vi "obstacle2.vi"(9 "Numeric":dbl, 10 "f":i32, 11 "Position in":T1) -> (0 "deliver":bool, 3 "Position out":T1)   [LabVIEW 2014]
uses:
  <vilib>/Utility/miscctls.llb/LVPositionTypeDef.ctl
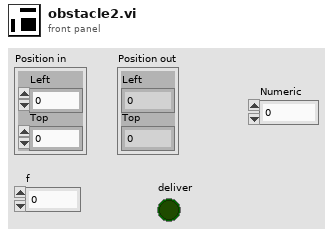
[diagram p1: front panel]
types:
  T1 = typedef "LVPositionTypeDef.ctl" = cluster{"Left":i32, "Top":i32}
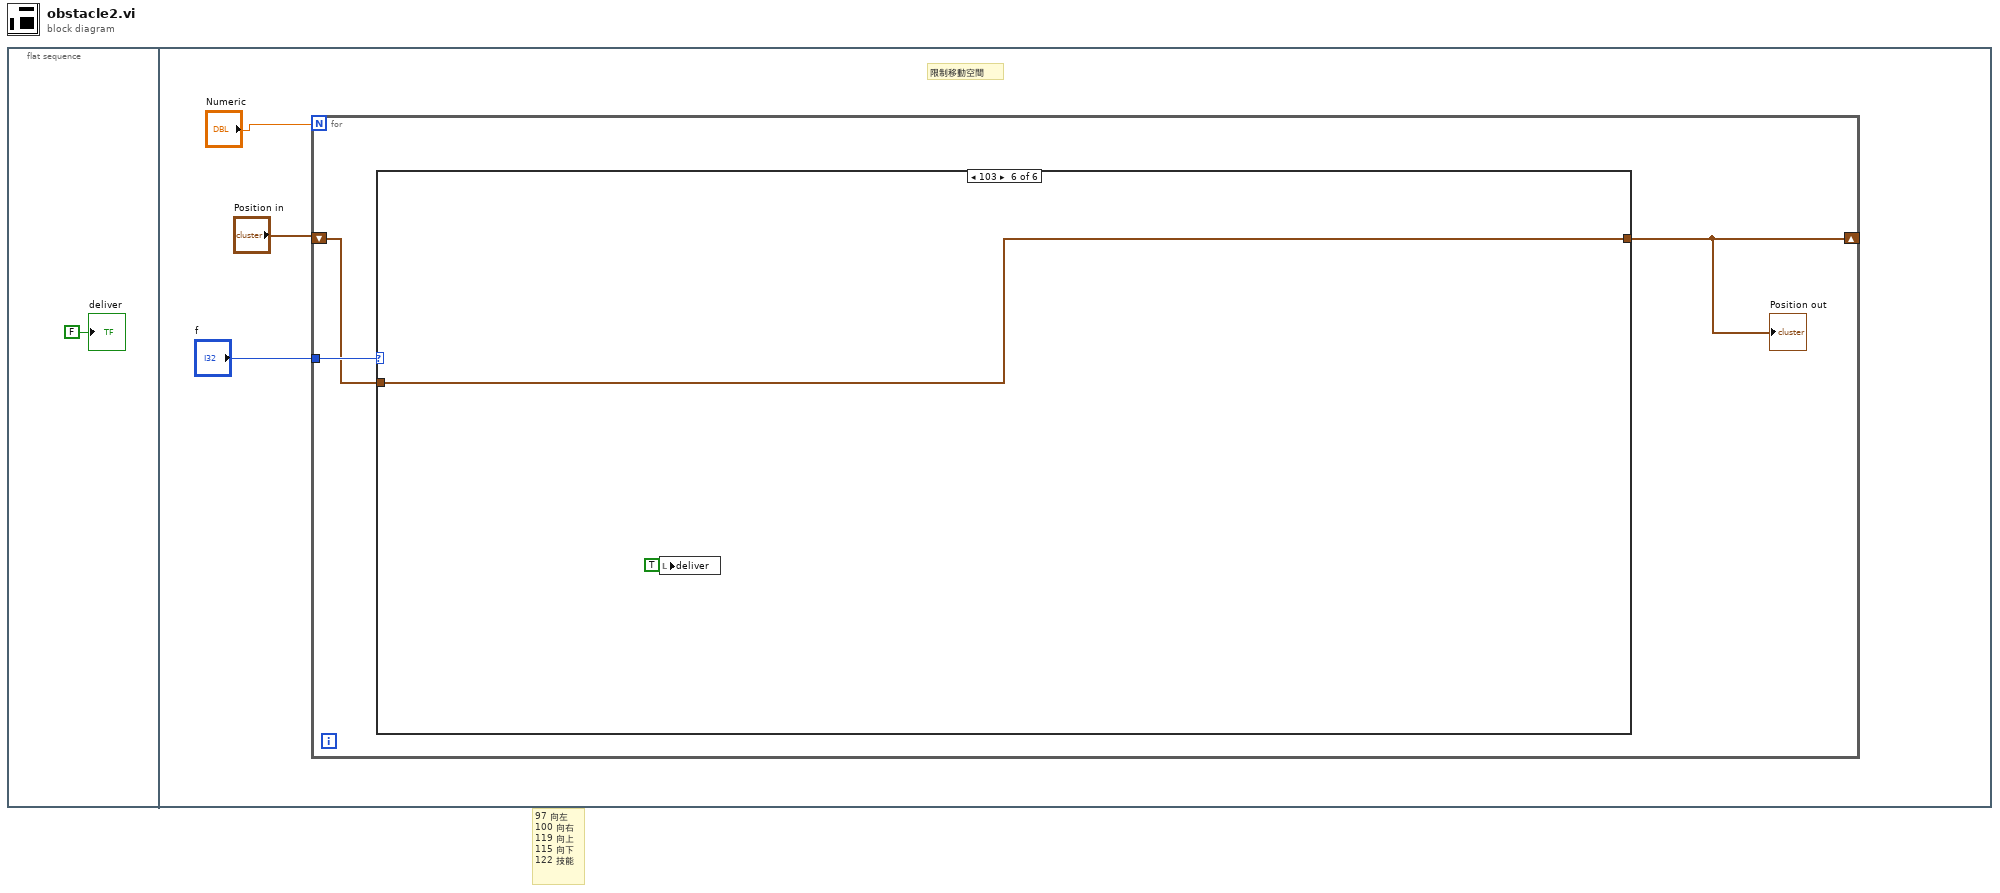
[diagram p0: block diagram]
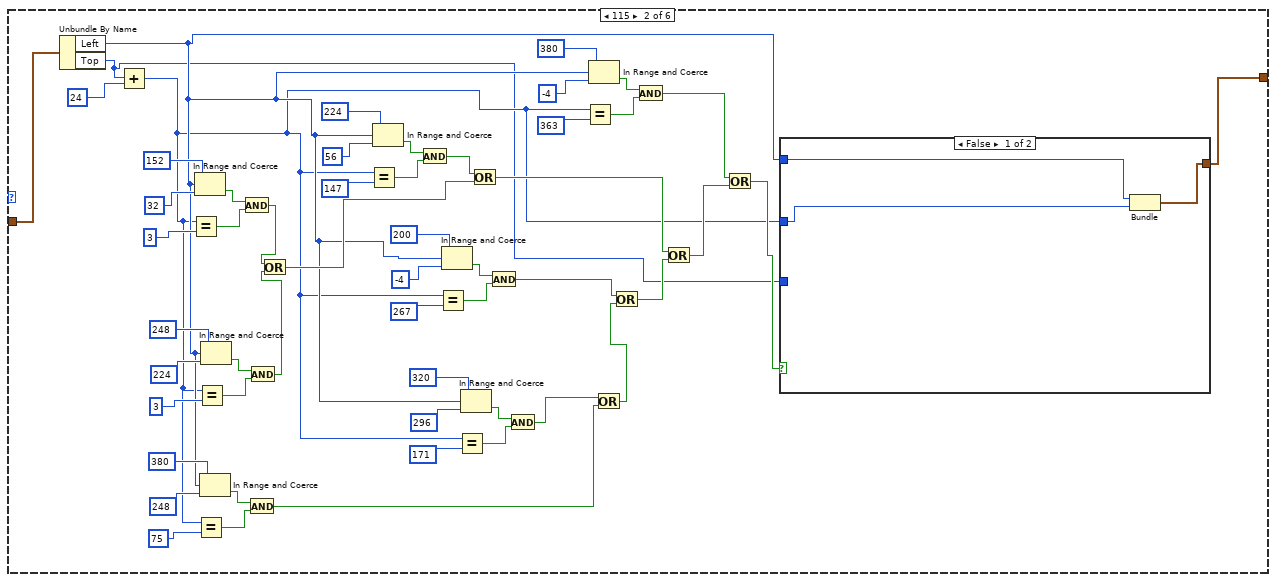
[diagram p3: hidden frame]
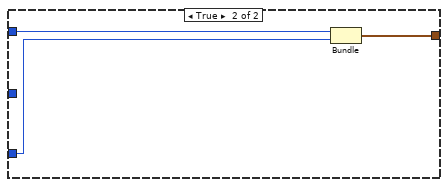
[diagram p4: hidden frame]
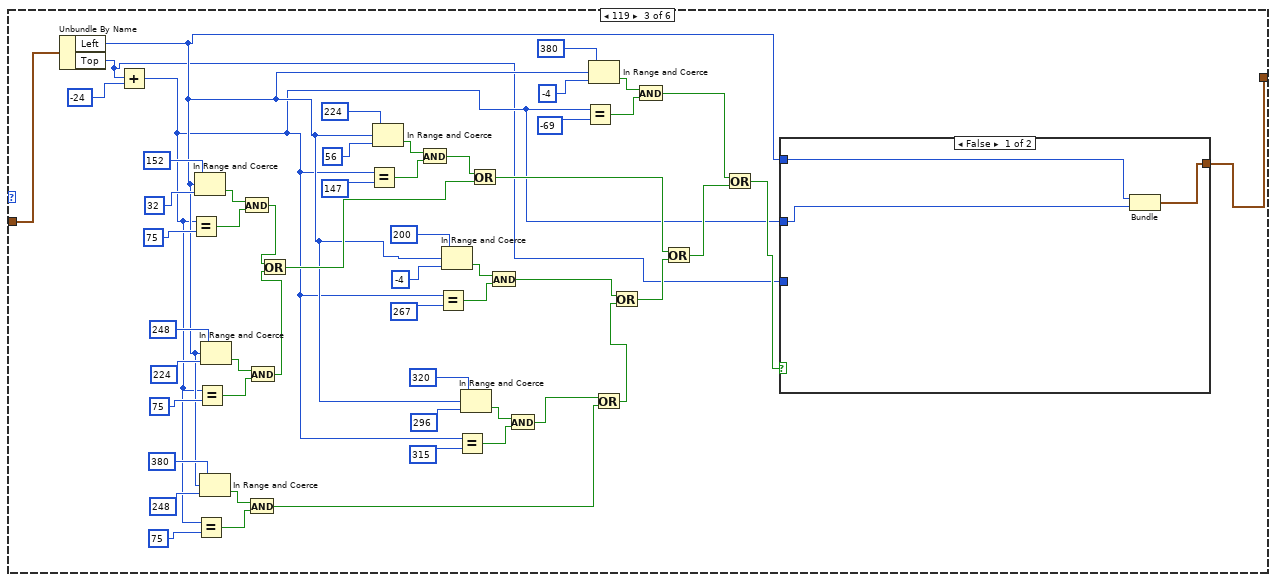
[diagram p5: hidden frame]
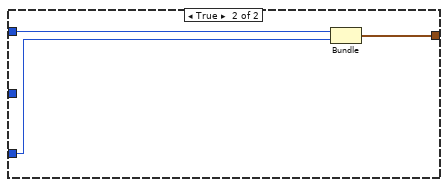
[diagram p6: hidden frame]
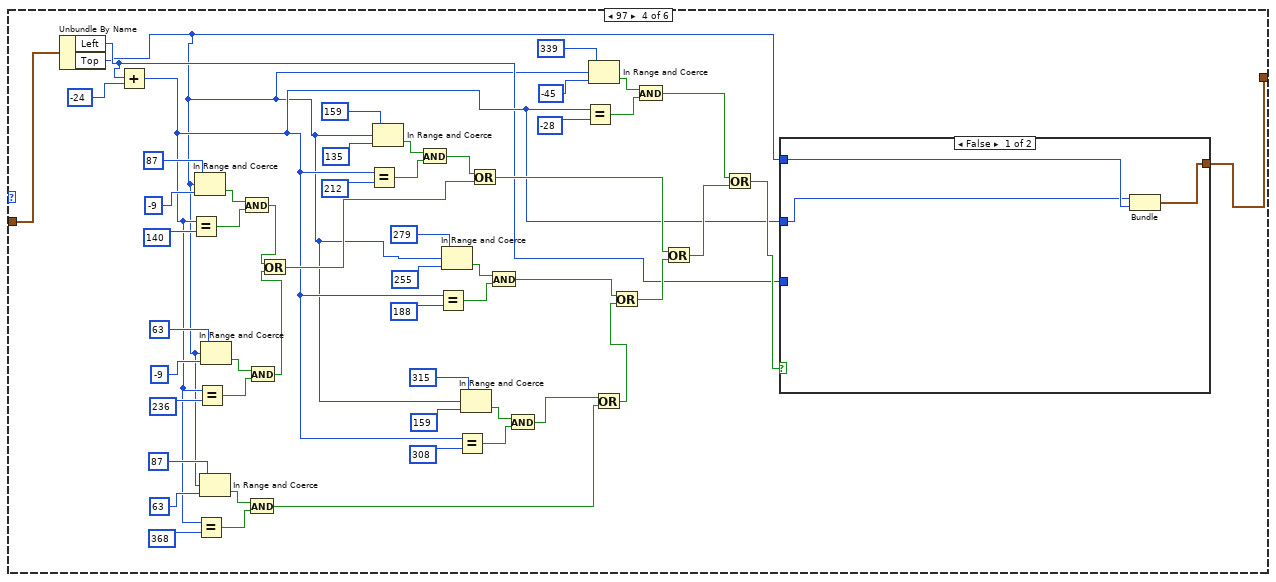
[diagram p7: hidden frame]
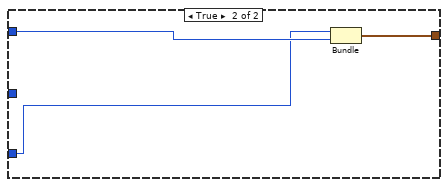
[diagram p8: hidden frame]
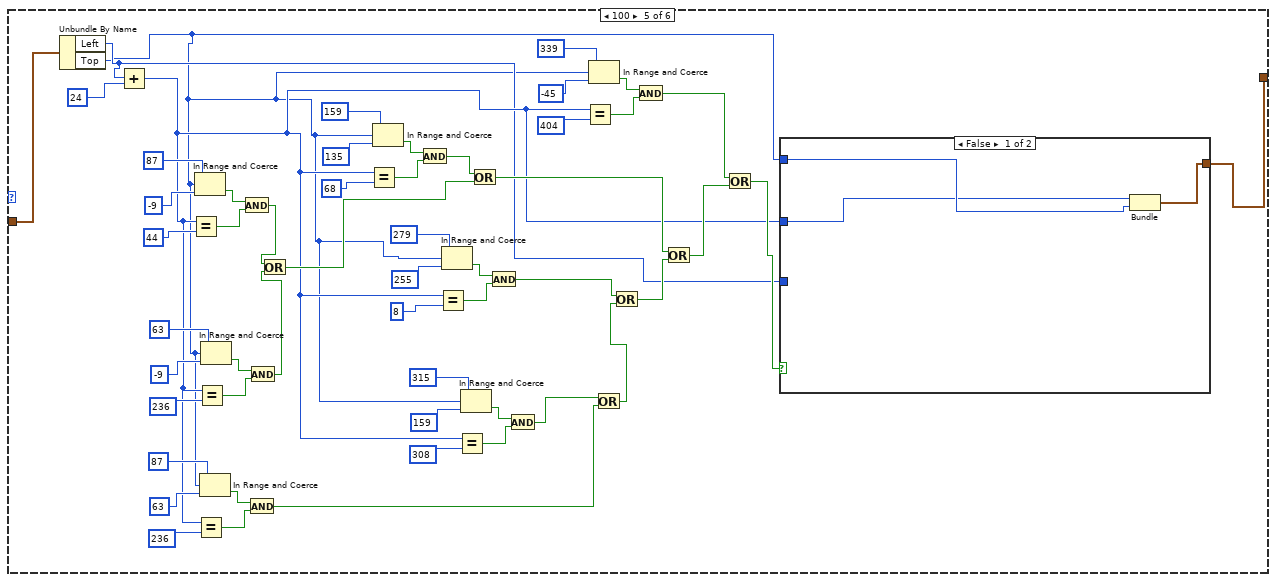
[diagram p9: hidden frame]
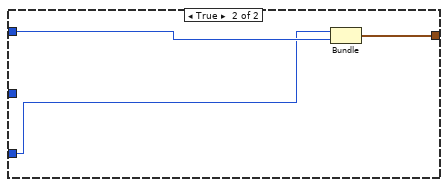
[diagram p10: hidden frame]
diagram:
  # "97 向左\n100 向右\n119 向上\n115 向下\n122 技能"
  n1 = flat-sequence {
    frame #0 {
      "deliver" <- FALSE ("skill")
    }
    frame #1 {
      # "限制移動空間"
      n2 = for {
        N: "Numeric" -> [_]
        tunnel: "f" -> [w7]
        shift-right: [w6] -> _
        shift-left: "Position in" -> [w5]
        n3 = case shown="103" w7 {
          tunnel: w5 -> [w8 w61 w121 w181 w241 w250]
          tunnel: [w8 w9 w120 w180 w240 w250] -> w6
          frame 0, Default {
          }
          frame 115 {
            n4 = Unbundle By Name(w61) -> ("Left"=w12:i32, "Top"=w10:i32)
            n5 = Add(x=w10, y=24) -> (x+y=w11:i32)
            n6 = Equal?(x=w11, y=3) -> (x = y?=w57:bool)
            n7 = In Range and Coerce(upper limit=152, x=w12, lower limit=32) -> (In Range?=w56:bool)  [unwired: 1 out]
            n8 = Equal?(x=w11, y=75) -> (x = y?=w47:bool)
            n9 = Equal?(x=w11, y=3) -> (x = y?=w52:bool)
            n10 = In Range and Coerce(upper limit=380, x=w12, lower limit=248) -> (In Range?=w46:bool)  [unwired: 1 out]
            n11 = In Range and Coerce(upper limit=248, x=w12, lower limit=224) -> (In Range?=w51:bool)  [unwired: 1 out]
            n12 = And(x=w56, y=w57) -> (x .and. y?=w30:bool)
            n13 = And(x=w46, y=w47) -> (x .and. y?=w26:bool)
            n14 = And(x=w51, y=w52) -> (x .and. y?=w29:bool)
            n15 = Or(x=w30, y=w29) -> (x .or. y?=w28:bool)
            n16 = Equal?(x=w11, y=147) -> (x = y?=w42:bool)
            n17 = In Range and Coerce(upper limit=224, x=w12, lower limit=56) -> (In Range?=w41:bool)  [unwired: 1 out]
            n18 = And(x=w41, y=w42) -> (x .and. y?=w27:bool)
            n19 = Equal?(x=w11, y=267) -> (x = y?=w37:bool)
            n20 = In Range and Coerce(upper limit=200, x=w12, lower limit=-4) -> (In Range?=w36:bool)  [unwired: 1 out]
            n21 = Equal?(x=w11, y=171) -> (x = y?=w32:bool)
            n22 = In Range and Coerce(upper limit=320, x=w12, lower limit=296) -> (In Range?=w31:bool)  [unwired: 1 out]
            n23 = Or(x=w27, y=w28) -> (x .or. y?=w21:bool)
            n24 = And(x=w36, y=w37) -> (x .and. y?=w24:bool)
            n25 = And(x=w31, y=w32) -> (x .and. y?=w25:bool)
            n26 = Equal?(x=w11, y=363) -> (x = y?=w17:bool)
            n27 = In Range and Coerce(upper limit=380, x=w12, lower limit=-4) -> (In Range?=w16:bool)  [unwired: 1 out]
            n28 = Or(x=w25, y=w26) -> (x .or. y?=w23:bool)
            n29 = Or(x=w24, y=w23) -> (x .or. y?=w22:bool)
            n30 = And(x=w16, y=w17) -> (x .and. y?=w15:bool)
            n31 = Or(x=w21, y=w22) -> (x .or. y?=w14:bool)
            n32 = Or(x=w15, y=w14) -> (x .or. y?=w13:bool)
            n33 = case shown="False" w13 {
              tunnel: w12 -> [w64 w67]
              tunnel: [w65 w68] -> w9
              tunnel: w11 -> [w63 _]
              tunnel: w10 -> [_ w66]
              frame False {
                n34 = Bundle("Left"=w64, w63) -> (w65:cluster{"Left":i32, i32})  [unwired: 1 in]
              }
              frame True {
                n35 = Bundle("Left"=w67, "Top"=w66) -> (w68:cluster{"Left":i32, "Top":i32})  [unwired: 1 in]
              }
            }
          }
          frame 119 {
            n36 = Unbundle By Name(w121) -> ("Left"=w71:i32, "Top"=w69:i32)
            n37 = Add(x=w69, y=-24) -> (x+y=w70:i32)
            n38 = Equal?(x=w70, y=75) -> (x = y?=w116:bool)
            n39 = In Range and Coerce(upper limit=152, x=w71, lower limit=32) -> (In Range?=w115:bool)  [unwired: 1 out]
            n40 = Equal?(x=w70, y=75) -> (x = y?=w106:bool)
            n41 = Equal?(x=w70, y=75) -> (x = y?=w111:bool)
            n42 = In Range and Coerce(upper limit=380, x=w71, lower limit=248) -> (In Range?=w105:bool)  [unwired: 1 out]
            n43 = In Range and Coerce(upper limit=248, x=w71, lower limit=224) -> (In Range?=w110:bool)  [unwired: 1 out]
            n44 = And(x=w115, y=w116) -> (x .and. y?=w89:bool)
            n45 = And(x=w105, y=w106) -> (x .and. y?=w85:bool)
            n46 = And(x=w110, y=w111) -> (x .and. y?=w88:bool)
            n47 = Or(x=w89, y=w88) -> (x .or. y?=w87:bool)
            n48 = Equal?(x=w70, y=147) -> (x = y?=w101:bool)
            n49 = In Range and Coerce(upper limit=224, x=w71, lower limit=56) -> (In Range?=w100:bool)  [unwired: 1 out]
            n50 = And(x=w100, y=w101) -> (x .and. y?=w86:bool)
            n51 = Equal?(x=w70, y=267) -> (x = y?=w96:bool)
            n52 = In Range and Coerce(upper limit=200, x=w71, lower limit=-4) -> (In Range?=w95:bool)  [unwired: 1 out]
            n53 = Equal?(x=w70, y=315) -> (x = y?=w91:bool)
            n54 = In Range and Coerce(upper limit=320, x=w71, lower limit=296) -> (In Range?=w90:bool)  [unwired: 1 out]
            n55 = Or(x=w86, y=w87) -> (x .or. y?=w80:bool)
            n56 = And(x=w95, y=w96) -> (x .and. y?=w83:bool)
            n57 = And(x=w90, y=w91) -> (x .and. y?=w84:bool)
            n58 = Equal?(x=w70, y=-69) -> (x = y?=w76:bool)
            n59 = In Range and Coerce(upper limit=380, x=w71, lower limit=-4) -> (In Range?=w75:bool)  [unwired: 1 out]
            n60 = Or(x=w84, y=w85) -> (x .or. y?=w82:bool)
            n61 = Or(x=w83, y=w82) -> (x .or. y?=w81:bool)
            n62 = And(x=w75, y=w76) -> (x .and. y?=w74:bool)
            n63 = Or(x=w80, y=w81) -> (x .or. y?=w73:bool)
            n64 = Or(x=w74, y=w73) -> (x .or. y?=w72:bool)
            n65 = case shown="False" w72 {
              tunnel: w71 -> [w124 w127]
              tunnel: [w125 w128] -> w120
              tunnel: w70 -> [w123 _]
              tunnel: w69 -> [_ w126]
              frame False {
                n66 = Bundle("Left"=w124, w123) -> (w125:cluster{"Left":i32, i32})  [unwired: 1 in]
              }
              frame True {
                n67 = Bundle("Left"=w127, "Top"=w126) -> (w128:cluster{"Left":i32, "Top":i32})  [unwired: 1 in]
              }
            }
          }
          frame 97 {
            n68 = Unbundle By Name(w181) -> ("Left"=w130:i32, "Top"=w129:i32)
            n69 = Add(x=w130, y=-24) -> (x+y=w131:i32)
            n70 = Equal?(x=w131, y=140) -> (x = y?=w176:bool)
            n71 = In Range and Coerce(upper limit=87, x=w129, lower limit=-9) -> (In Range?=w175:bool)  [unwired: 1 out]
            n72 = Equal?(x=w131, y=368) -> (x = y?=w166:bool)
            n73 = Equal?(x=w131, y=236) -> (x = y?=w171:bool)
            n74 = In Range and Coerce(upper limit=87, x=w129, lower limit=63) -> (In Range?=w165:bool)  [unwired: 1 out]
            n75 = In Range and Coerce(upper limit=63, x=w129, lower limit=-9) -> (In Range?=w170:bool)  [unwired: 1 out]
            n76 = And(x=w175, y=w176) -> (x .and. y?=w149:bool)
            n77 = And(x=w165, y=w166) -> (x .and. y?=w145:bool)
            n78 = And(x=w170, y=w171) -> (x .and. y?=w148:bool)
            n79 = Or(x=w149, y=w148) -> (x .or. y?=w147:bool)
            n80 = Equal?(x=w131, y=212) -> (x = y?=w161:bool)
            n81 = In Range and Coerce(upper limit=159, x=w129, lower limit=135) -> (In Range?=w160:bool)  [unwired: 1 out]
            n82 = And(x=w160, y=w161) -> (x .and. y?=w146:bool)
            n83 = Equal?(x=w131, y=188) -> (x = y?=w156:bool)
            n84 = In Range and Coerce(upper limit=279, x=w129, lower limit=255) -> (In Range?=w155:bool)  [unwired: 1 out]
            n85 = Equal?(x=w131, y=308) -> (x = y?=w151:bool)
            n86 = In Range and Coerce(upper limit=315, x=w129, lower limit=159) -> (In Range?=w150:bool)  [unwired: 1 out]
            n87 = Or(x=w146, y=w147) -> (x .or. y?=w140:bool)
            n88 = And(x=w155, y=w156) -> (x .and. y?=w143:bool)
            n89 = And(x=w150, y=w151) -> (x .and. y?=w144:bool)
            n90 = Equal?(x=w131, y=-28) -> (x = y?=w136:bool)
            n91 = In Range and Coerce(upper limit=339, x=w129, lower limit=-45) -> (In Range?=w135:bool)  [unwired: 1 out]
            n92 = Or(x=w144, y=w145) -> (x .or. y?=w142:bool)
            n93 = Or(x=w143, y=w142) -> (x .or. y?=w141:bool)
            n94 = And(x=w135, y=w136) -> (x .and. y?=w134:bool)
            n95 = Or(x=w140, y=w141) -> (x .or. y?=w133:bool)
            n96 = Or(x=w134, y=w133) -> (x .or. y?=w132:bool)
            n97 = case shown="False" w132 {
              tunnel: w129 -> [w184 w187]
              tunnel: [w185 w188] -> w180
              tunnel: w131 -> [w183 _]
              tunnel: w130 -> [_ w186]
              frame False {
                n98 = Bundle(w183, "Top"=w184) -> (w185:cluster{i32, "Top":i32})  [unwired: 1 in]
              }
              frame True {
                n99 = Bundle("Left"=w186, "Top"=w187) -> (w188:cluster{"Left":i32, "Top":i32})  [unwired: 1 in]
              }
            }
          }
          frame 100 {
            n100 = Unbundle By Name(w241) -> ("Left"=w190:i32, "Top"=w189:i32)
            n101 = Add(x=w190, y=24) -> (x+y=w191:i32)
            n102 = Equal?(x=w191, y=44) -> (x = y?=w236:bool)
            n103 = In Range and Coerce(upper limit=87, x=w189, lower limit=-9) -> (In Range?=w235:bool)  [unwired: 1 out]
            n104 = Equal?(x=w191, y=236) -> (x = y?=w226:bool)
            n105 = Equal?(x=w191, y=236) -> (x = y?=w231:bool)
            n106 = In Range and Coerce(upper limit=87, x=w189, lower limit=63) -> (In Range?=w225:bool)  [unwired: 1 out]
            n107 = In Range and Coerce(upper limit=63, x=w189, lower limit=-9) -> (In Range?=w230:bool)  [unwired: 1 out]
            n108 = And(x=w235, y=w236) -> (x .and. y?=w209:bool)
            n109 = And(x=w225, y=w226) -> (x .and. y?=w205:bool)
            n110 = And(x=w230, y=w231) -> (x .and. y?=w208:bool)
            n111 = Or(x=w209, y=w208) -> (x .or. y?=w207:bool)
            n112 = Equal?(x=w191, y=68) -> (x = y?=w221:bool)
            n113 = In Range and Coerce(upper limit=159, x=w189, lower limit=135) -> (In Range?=w220:bool)  [unwired: 1 out]
            n114 = And(x=w220, y=w221) -> (x .and. y?=w206:bool)
            n115 = Equal?(x=w191, y=8) -> (x = y?=w216:bool)
            n116 = In Range and Coerce(upper limit=279, x=w189, lower limit=255) -> (In Range?=w215:bool)  [unwired: 1 out]
            n117 = Equal?(x=w191, y=308) -> (x = y?=w211:bool)
            n118 = In Range and Coerce(upper limit=315, x=w189, lower limit=159) -> (In Range?=w210:bool)  [unwired: 1 out]
            n119 = Or(x=w206, y=w207) -> (x .or. y?=w200:bool)
            n120 = And(x=w215, y=w216) -> (x .and. y?=w203:bool)
            n121 = And(x=w210, y=w211) -> (x .and. y?=w204:bool)
            n122 = Equal?(x=w191, y=404) -> (x = y?=w196:bool)
            n123 = In Range and Coerce(upper limit=339, x=w189, lower limit=-45) -> (In Range?=w195:bool)  [unwired: 1 out]
            n124 = Or(x=w204, y=w205) -> (x .or. y?=w202:bool)
            n125 = Or(x=w203, y=w202) -> (x .or. y?=w201:bool)
            n126 = And(x=w195, y=w196) -> (x .and. y?=w194:bool)
            n127 = Or(x=w200, y=w201) -> (x .or. y?=w193:bool)
            n128 = Or(x=w194, y=w193) -> (x .or. y?=w192:bool)
            n129 = case shown="False" w192 {
              tunnel: w189 -> [w244 w247]
              tunnel: [w245 w248] -> w240
              tunnel: w191 -> [w243 _]
              tunnel: w190 -> [_ w246]
              frame False {
                n130 = Bundle(w243, "Top"=w244) -> (w245:cluster{i32, "Top":i32})  [unwired: 1 in]
              }
              frame True {
                n131 = Bundle("Left"=w246, "Top"=w247) -> (w248:cluster{"Left":i32, "Top":i32})  [unwired: 1 in]
              }
            }
          }
          frame 103 {
            n132 = local write "deliver"(TRUE ("skill")) -> ()
          }
        }
        "Position out" <- w6
      }
    }
  }
